vi "Serial Data Recieve.vi"(1 "Stoped":bool, 10 "VISA resource name":refnum<visa-resource-name>) -> (0 "array":string[](array[string]), 2 "OK":bool, 3 "leak":string)   [LabVIEW 2015]
uses:
  <vilib>/Instr/_visa.llb/VISA Configure Serial Port (Instr).vi
panel:
  in  "Stoped 2":bool
  in  "index":i32=3
  out "read string":string
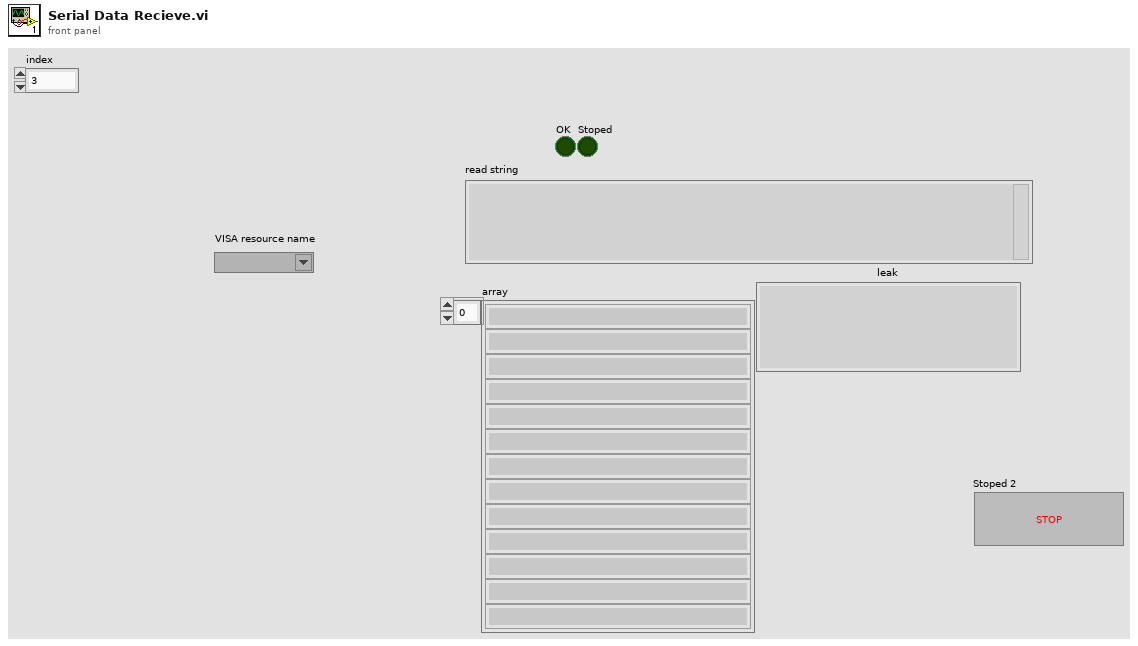
[diagram p1: front panel]
types:
  T1 = cluster{"Barcode Scanner 2":refnum<visa-resource-name>, "baud rate":u32, "data bits":u16, "parity":enum16{"None", "Odd", "Even", "Mark", "Space"}, "stop bits":u16, "flow control":u16}
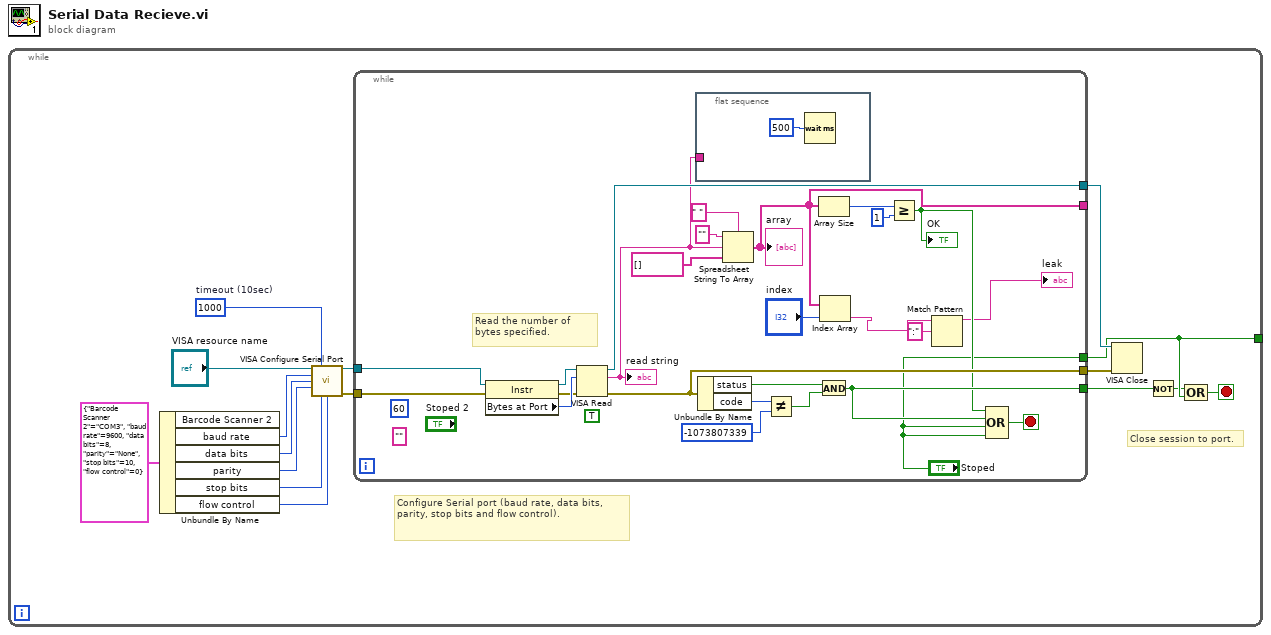
[diagram p0: block diagram]
diagram:
  n1 = while {
    tunnel: [w3] -> _
    stop <- w1 stop-if-true
    w14 = u32 1000  # timeout (10sec)
    # "Close session to port."
    # "Configure Serial port (baud rate, data bits, parity, stop bits and flow control)."
    n2 = Unbundle By Name(T1 {"Barcode Scanner 2"="COM3", "baud rate"=9600, "data bits"=8, "parity"=enum."None", "stop bits"=10, "flow control"=0} ("Serial Parameters")) -> ("baud rate"=w10:u32, "data bits"=w9:u16, "parity"=w8:enum16{"None", "Odd", "Even", "Mark", "Space"}, "stop bits"=w7:u16, "flow control"=w6:u16)  [unwired: 1 out]
    n3 = call-poly "VISA Configure Serial Port"("VISA resource name"="VISA resource name", "timeout (10sec)"=w14, "baud rate (9600)"=w10, "data bits (8)"=w9, "parity (0:none)"=w8, "stop bits (10: 1 bit)"=w7, "flow control (0:none)"=w6) -> ("VISA resource name out"=w13:refnum<visa-resource-name>, "error out"=w12:errorcluster)  [unwired: 2 in, 5 out]
    n4 = while {
      tunnel: [w41] -> w16
      tunnel: [w42] -> w15
      tunnel: w12 -> [w26]
      tunnel: w13 -> [w30]
      tunnel: [w35] -> w5
      tunnel: ["Stoped"] -> w3
      tunnel: [w21] -> _
      stop <- w40 stop-if-true
      (unwired) ""
      (unwired) TRUE ("OK")
      (unwired) u32 60 ("byte count")
      # "Read the number of bytes specified."
      n5 = property class="Instr"(reference=w30, error in=w26) -> (reference out=w28:refnum<visa-resource-name>, error out=w27:errorcluster, "Bytes at Port"=w29:u32)
      n6 = VISA Read(VISA resource name=w28, byte count=w29, error in (no error)=w27) -> (VISA resource name out=w42:refnum<visa-resource-name>, read buffer=w22:string, error out=w41:errorcluster)  [unwired: 1 out]
      "read string" <- w22
      n7 = flat-sequence {
        tunnel: w22 -> [_]
        frame #0 {
          n8 = Wait (ms)(milliseconds to wait=u32 500) -> ()  [unwired: 1 out]
        }
      }
      n9 = Unbundle By Name(w41) -> ("status"=w39:bool, "code"=w38:i32)
      n10 = Spreadsheet String To Array(delimiter (Tab)=" ", format string="", spreadsheet string=w22, array type (2D Dbl)=string[] []) -> (array=w21:string[])
      "array" <- w21
      n11 = Not Equal?(x=w38, y=-1073807339 ("code")) -> (x != y?=w36:bool)
      n12 = Array Size(array=w21) -> (size(s)=w25:i32)
      n13 = And(x=w39, y=w36) -> (x .and. y?=w35:bool)
      n14 = Index Array(array=w21, index="index") -> (element=w19:string)
      n15 = Greater Or Equal?(x=w25, y=1) -> (x >= y?=w23:bool)
      "OK" <- w23
      n16 = Match Pattern(string=w19, regular expression=":") -> (before substring=→"leak":string)  [unwired: 1 in, 3 out]
      n17 = Compound Arithmetic op=OR(w23, w35, "Stoped", "Stoped") -> (w40:bool)
    }
    n18 = VISA Close(VISA resource name=w15, error in (no error)=w16) -> ()  [unwired: 1 out]
    n19 = Not(x=w5) -> (.not. x?=w2:bool)
    n20 = Compound Arithmetic op=OR(w2, w3) -> (w1:bool)
  }
